vi "uA__daq_Get_diana_uA_Vbat_for_reading.vi"(8 "error in (no error)":errorcluster, 10 "Coef":dbl, 11 "Refnum in":refnum<k21>) -> (0 "error out":errorcluster, 1 "Vbat":dbl, 2 "UA":waveform(dbl)(graph), 3 "uA Current":dbl, 5 "task out":refnum<k21>)   [LabVIEW 2015]
uses:
  <vilib>/DAQmx/read.llb/DAQmx Read (Analog 1D Wfm NChan NSamp).vi
  <vilib>/DAQmx/miscellaneous.llb/DAQmx Fill In Error Info.vi
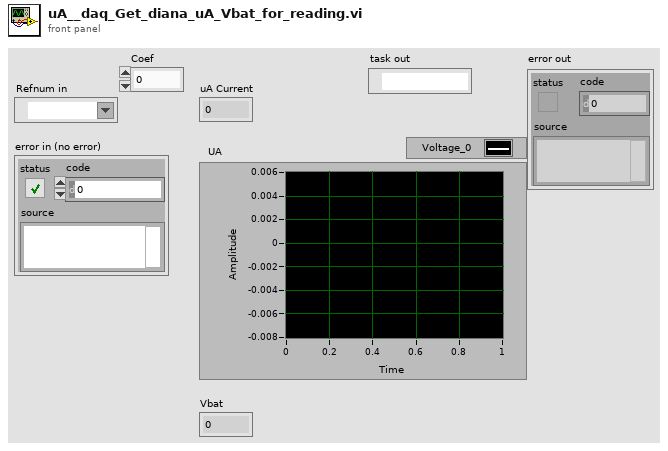
[diagram p1: front panel]
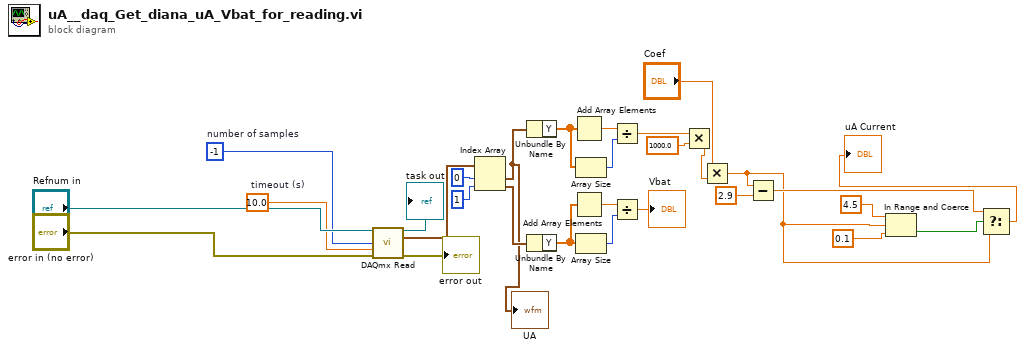
[diagram p0: block diagram]
diagram:
  w15 = 10.0  # timeout (s)
  w14 = -1  # number of samples
  n1 = call-poly <vilib>:"DAQmx Read.vi"("task/channels in"="Refnum in", "number of samples per channel"=w14, "timeout"=w15, "error in"="error in (no error)") -> ("task out"=→"task out":refnum<k21>, "data"=w18:waveform(dbl)[], "error out"=→"error out":errorcluster)  [unwired: 9 in]
  n2 = Index Array(array=w18, index #1=0 ("index"), index #2=1 ("index")) -> (element #1=w9:waveform(dbl), element #2=w10:waveform(dbl))
  "UA" <- w9
  n3 = Unbundle By Name(w9) -> ("Y"=w22:dbl[])
  n4 = Unbundle By Name(w10) -> ("Y"=w27:dbl[])
  n5 = Add Array Elements(numeric array=w22) -> (sum=w21:dbl)
  n6 = Add Array Elements(numeric array=w27) -> (sum=w28:dbl)
  n7 = Array Size(array=w22) -> (size(s)=w23:i32)
  n8 = Array Size(array=w27) -> (size(s)=w26:i32)
  n9 = Divide(x=w21, y=w23) -> (x/y=w24:dbl)
  n10 = Divide(x=w28, y=w26) -> (x/y=→"Vbat":dbl)
  n11 = Multiply(x=w24, y=1000.0) -> (x*y=w12:dbl)
  n12 = Multiply(x="Coef", y=w12) -> (x*y=w4:dbl)
  n13 = Subtract(x=w4, y=2.9) -> (x-y=w6:dbl)
  n14 = In Range and Coerce(upper limit=4.5, x=w4, lower limit=0.1 ("y")) -> (In Range?=w7:bool)  [unwired: 1 out]
  n15 = Select(t=w6, s=w7, f=w4) -> (s? t:f=→"uA Current":dbl)
